vi "EnableDisableCtls.vi"(10 "Ctls array":refnum<vi>[](array[refnum]), 11 "Enable/Disable":T1(ring)) -> ()   [LabVIEW 2020]
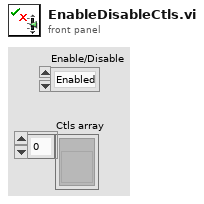
[diagram p1: front panel]
types:
  T1 = enum8{"Enabled", "Disabled", "Disabled and Grayed Out"}
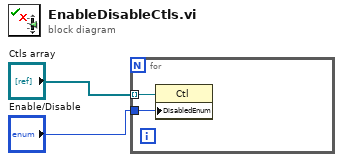
[diagram p0: block diagram]
diagram:
  n1 = for {
    tunnel: "Ctls array" -> [w3] mode=indexing
    tunnel: "Enable/Disable" -> [w4]
    n2 = property class="Ctl"(reference=w3, "DisabledEnum"=w4) -> ()  [unwired: 1 in, 2 out]
  }
